vi "Multi Channel Stream.vi"() -> ()   [LabVIEW 2020]
uses:
  Channel/Channel.lvclass
  Stream/Stream.lvclass
  <vilib>/Utility/config.llb/NI_LVConfig.lvlib
  <vilib>/Utility/config.llb/Read Key (String).vi
panel:
  out "appended path":path
  in  "Stop":bool
  out "error out":errorcluster
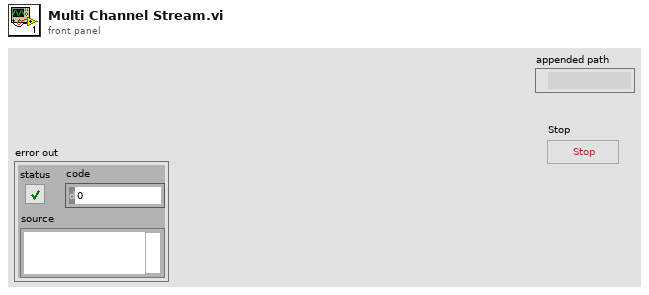
[diagram p1: front panel]
types:
  T1 = typedef "NI_LVConfig.lvlib/Config Data RefNum.ctl" = refnum<k1>
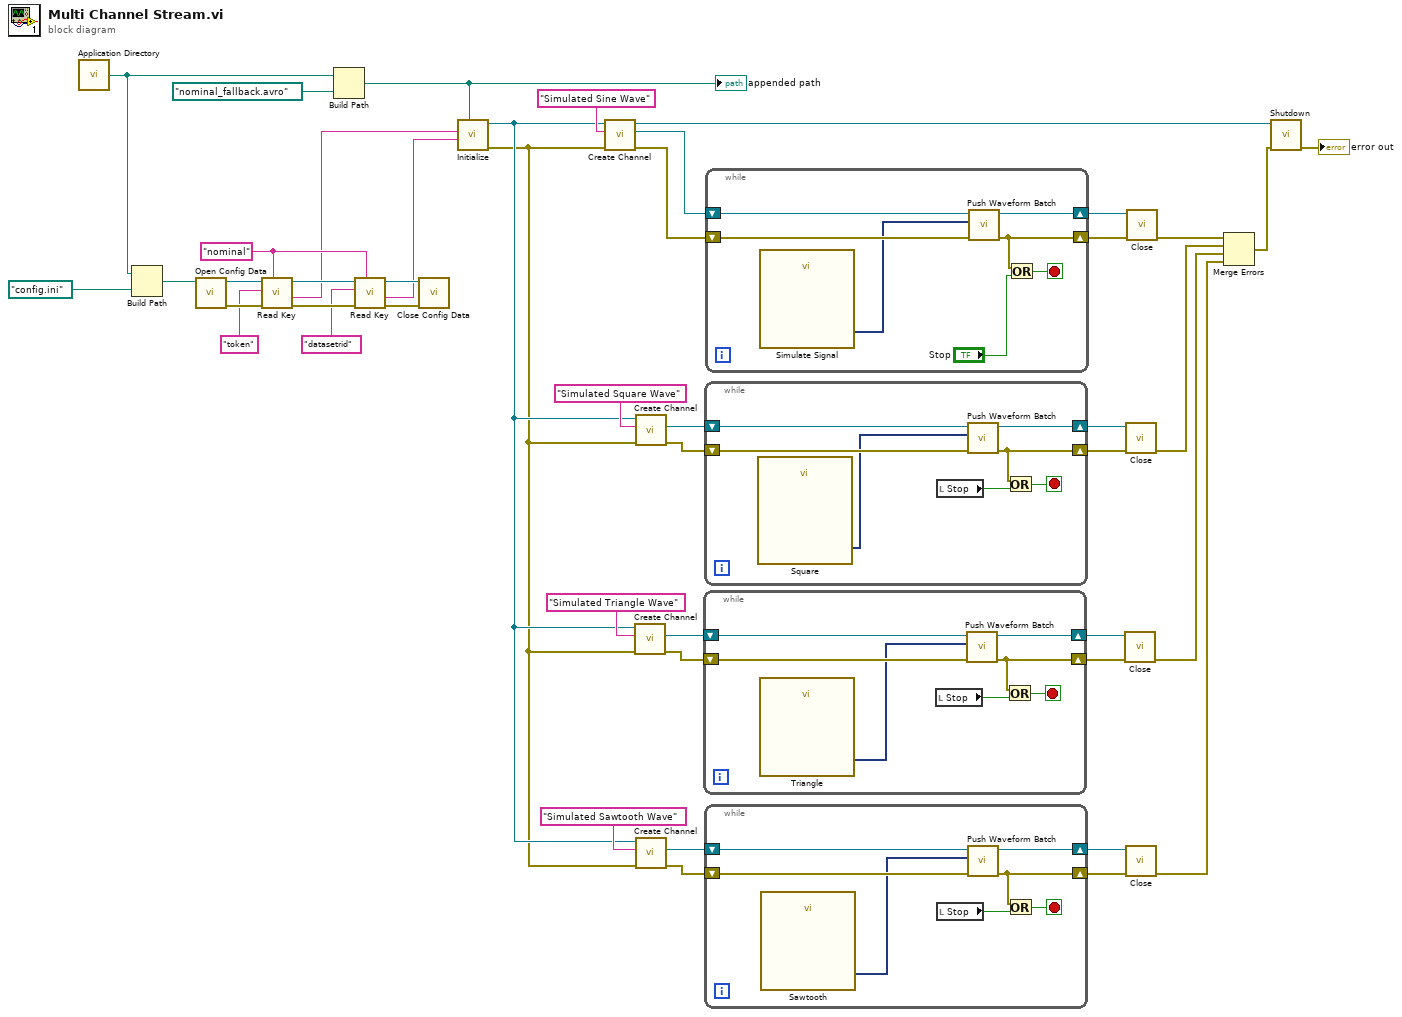
[diagram p0: block diagram]
diagram:
  w4 = "nominal" ("section")
  n1 = call <vilib>:"Application Directory.vi"() -> ("Application Directory"=w1:path)
  n2 = Build Path(base path=w1, name or relative path=path "config.ini") -> (appended path=w13:path)
  n3 = call <vilib>:"Open Config Data.vi"("configuration file path"=w13) -> ("error out"=w7:errorcluster, "refnum"=w12:T1)  [unwired: 8 in, 1 out]
  n4 = call-poly <vilib>:"Read Key.vi"("section"=w4, "error in (no error)"=w7, "key"="token", "refnum"=w12) -> ("error out"=w8:errorcluster, "value"=w3:string, "refnum out"=w11:T1)  [unwired: 4 in, 1 out]
  n5 = Build Path(base path=w1, name or relative path=path "nominal_fallback.avro") -> (appended path=w37:path)
  "appended path" <- w37
  n6 = call-poly <vilib>:"Read Key.vi"("section"=w4, "error in (no error)"=w8, "key"="datasetrid", "refnum"=w11) -> ("error out"=w9:errorcluster, "value"=w2:string, "refnum out"=w10:T1)  [unwired: 4 in, 1 out]
  n7 = call <vilib>:"Close Config Data.vi"("error in (no error)"=w9, "refnum"=w10) -> ()  [unwired: 8 in, 2 out]
  n8 = call "Initialize.vi"("Fallback File Path"=w37, "Dataset RID"=w2, "Token"=w3) -> ("error out"=w15:errorcluster, "Nominal Streaming out"=w17:refnum<class "Stream.lvclass">)  [unwired: 7 in]
  n9 = call "Create Channel.vi"("error in (no error)"=w15, "Channel Name"="Simulated Sine Wave", "Nominal Streaming in"=w17) -> ("error out"=w42:errorcluster, "Channel"=w43:refnum<class "Channel.lvclass">, "Nominal Streaming out"=w41:refnum<class "Stream.lvclass">)  [unwired: 6 in]
  n10 = call "Create Channel.vi"("error in (no error)"=w15, "Channel Name"="Simulated Triangle Wave", "Nominal Streaming in"=w17) -> ("error out"=w27:errorcluster, "Channel"=w26:refnum<class "Channel.lvclass">)  [unwired: 6 in, 1 out]
  n11 = call "Create Channel.vi"("error in (no error)"=w15, "Channel Name"="Simulated Square Wave", "Nominal Streaming in"=w17) -> ("error out"=w34:errorcluster, "Channel"=w35:refnum<class "Channel.lvclass">)  [unwired: 6 in, 1 out]
  n12 = call "Create Channel.vi"("error in (no error)"=w15, "Channel Name"="Simulated Sawtooth Wave", "Nominal Streaming in"=w17) -> ("error out"=w20:errorcluster, "Channel"=w21:refnum<class "Channel.lvclass">)  [unwired: 6 in, 1 out]
  n13 = while {
    shift-right: [w52] -> w25
    shift-left: w26 -> [w51]
    shift-right: [w50] -> w28
    shift-left: w27 -> [w48]
    stop <- w49 stop-if-true
    n14 = call "Triangle"() -> ("Triangle"=w46:dynamicdata)  [unwired: 14 in, 1 out]
    n15 = local read "Stop"() -> (w47:bool)
    n16 = call "Push Waveform Batch.vi"("error in (no error)"=w48, "Waveform"=w46, "Channel in"=w51) -> ("error out"=w50:errorcluster, "Channel out"=w52:refnum<class "Channel.lvclass">)  [unwired: 7 in]
    n17 = Or(x=w50, y=w47) -> (x .or. y?=w49:bool)
  }
  n18 = while {
    shift-right: [w59] -> w36
    shift-left: w35 -> [w58]
    shift-right: [w57] -> w33
    shift-left: w34 -> [w55]
    stop <- w56 stop-if-true
    n19 = call "Square"() -> ("Square"=w53:dynamicdata)  [unwired: 14 in, 1 out]
    n20 = local read "Stop"() -> (w54:bool)
    n21 = call "Push Waveform Batch.vi"("error in (no error)"=w55, "Waveform"=w53, "Channel in"=w58) -> ("error out"=w57:errorcluster, "Channel out"=w59:refnum<class "Channel.lvclass">)  [unwired: 7 in]
    n22 = Or(x=w57, y=w54) -> (x .or. y?=w56:bool)
  }
  n23 = while {
    shift-right: [w66] -> w22
    shift-left: w21 -> [w65]
    shift-right: [w64] -> w19
    shift-left: w20 -> [w62]
    stop <- w63 stop-if-true
    n24 = call "Sawtooth"() -> ("Sawtooth"=w60:dynamicdata)  [unwired: 14 in, 1 out]
    n25 = local read "Stop"() -> (w61:bool)
    n26 = call "Push Waveform Batch.vi"("error in (no error)"=w62, "Waveform"=w60, "Channel in"=w65) -> ("error out"=w64:errorcluster, "Channel out"=w66:refnum<class "Channel.lvclass">)  [unwired: 7 in]
    n27 = Or(x=w64, y=w61) -> (x .or. y?=w63:bool)
  }
  n28 = while {
    shift-right: [w73] -> w44
    shift-left: w43 -> [w72]
    shift-right: [w71] -> w40
    shift-left: w42 -> [w68]
    stop <- w70 stop-if-true
    n29 = call "Simulate Signal"() -> ("Sine"=w67:dynamicdata)  [unwired: 14 in, 1 out]
    n30 = call "Push Waveform Batch.vi"("error in (no error)"=w68, "Waveform"=w67, "Channel in"=w72) -> ("error out"=w71:errorcluster, "Channel out"=w73:refnum<class "Channel.lvclass">)  [unwired: 7 in]
    n31 = Or(x=w71, y="Stop") -> (x .or. y?=w70:bool)
  }
  n32 = call "Close.vi"("error in (no error)"=w28, "Channel in"=w25) -> ("error out"=w23:errorcluster)  [unwired: 9 in]
  n33 = call "Close.vi"("error in (no error)"=w33, "Channel in"=w36) -> ("error out"=w24:errorcluster)  [unwired: 9 in]
  n34 = call "Close.vi"("error in (no error)"=w19, "Channel in"=w22) -> ("error out"=w16:errorcluster)  [unwired: 9 in]
  n35 = call "Close.vi"("error in (no error)"=w40, "Channel in"=w44) -> ("error out"=w31:errorcluster)  [unwired: 9 in]
  n36 = Merge Errors(w31, w24, w23, w16) -> (w30:errorcluster)
  n37 = call "Shutdown.vi"("error in (no error)"=w30, "Nominal Streaming in"=w41) -> ("error out"=→"error out":errorcluster)  [unwired: 8 in, 1 out]
